vi "Validate Line Configuration Test.vi"() -> (2 "Pass":bool)   [LabVIEW 2015, in "Modbus Tests.lvlib"]
doc: "Test validate line configuration.vi to ensure that it catches all unique cases in which a channel should not be added to an existing configuration."
uses:
  Modbus Tests.lvlib
  editor node/table line.ctl
  module/module channel/Modbus Module Channel.lvclass
  <vilib>/NI/Tag Bus/tag/Data Type.ctl
  module/module channel/data bank type.ctl
  <vilib>/NI/Tag Bus Module Framework/channel/channel classification.ctl
  module/configuration/Modbus Module configuration.lvclass
  <vilib>/NI/Tag Bus/tag/tag descriptor.lvclass/tag descriptor.ctl
  module/module channel/Modbus Module Channel.lvclass/Modbus Module Channel.ctl
  <vilib>/NI/Tag Bus Module Framework/channel/TBM channel.lvclass/TBM channel.ctl
  <vilib>/NI/Tag Bus/tag/write data type.vi
  <vilib>/NI/Tag Bus/tag/write tag name.vi
  module/module channel/Write modbus type.vi
  module/module channel/Write starting address.vi
  module/module channel/Write subindex (bool).vi
  <vilib>/NI/Tag Bus Module Framework/channel/Write channel classification.vi
  editor node/Modbus Module editor node.lvclass
  <vilib>/NI/Tag Bus/tag/tag descriptor.lvclass
  <vilib>/NI/Tag Bus Module Framework/channel/TBM channel.lvclass
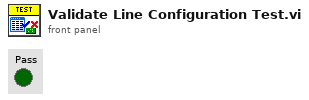
[diagram p1: front panel]
types:
  T1 = typedef "Modbus Module Channel.lvclass/data bank type.ctl" = enum16{"Coils", "Discrete Inputs", "Input Registers", "Holding Registers"}
  T2 = typedef "tag bus.lvlib/tag descriptor.lvclass/Data Type.ctl" = enum16{"Double", "Single", "I64", "I32", "I16", "I8", "U64", "U32", "U16", "U8", "Boolean", "String", "Array of Double", "Array of Single", "Array of I64", "Array of I32", "Array of I16", "Array of I8", "Array of U64", "Array of U32", "Array of U16", "Array of U8", "Array of Boolean", "Array of String"}
  T3 = typedef "TBM channel.lvclass/channel classification.ctl" = enum16{"input data", "output data", "processing parameter", "processing result"}
  T4 = typedef "Modbus Module editor node.lvclass/table line.ctl" = cluster{"mbchan":refnum<class "Modbus Module Channel.lvclass">, "tag name":string}
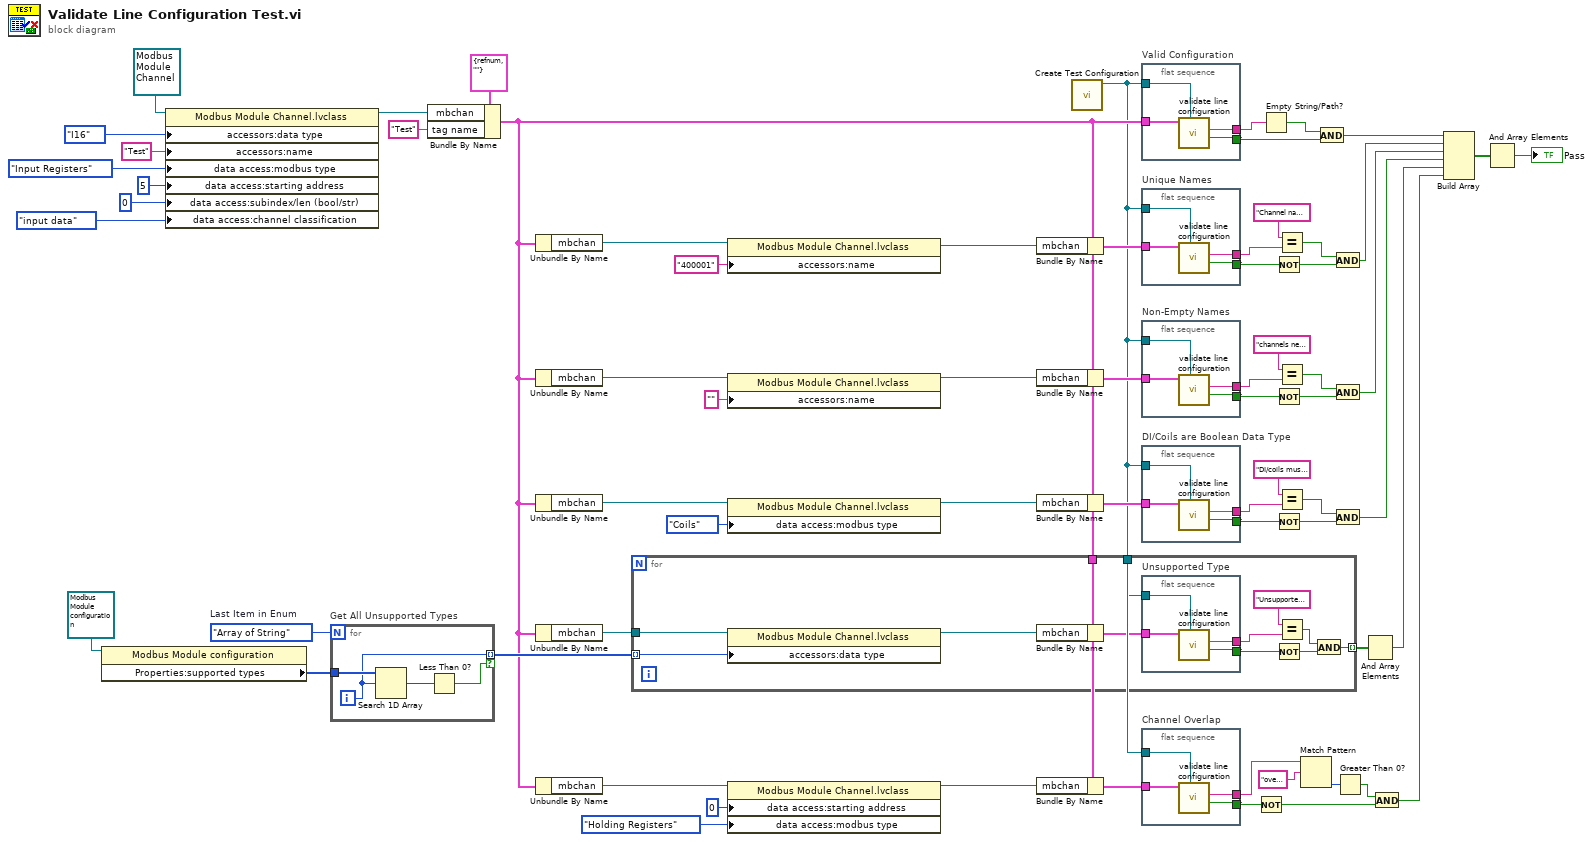
[diagram p0: block diagram]
diagram:
  w17 = Data_Type."Array of String"  # Last Item in Enum
  n1 = property class="Modbus Module configuration"(reference=refnum<class "Modbus Module configuration.lvclass"> refnum ("Modbus Module configuration")) -> ("Properties:supported types"=w18:T2[])  [unwired: 1 in, 2 out]
  n2 = property class="Modbus Module Channel.lvclass"(reference=refnum<class "Modbus Module Channel.lvclass"> refnum ("mbchan"), "accessors:data type"=Data_Type."I16" ("data type"), "accessors:name"="Test" ("name"), "data access:modbus type"=data_bank_type."Input Registers" ("modbus type"), "data access:starting address"=u16 5 ("starting address"), "data access:subindex/len (bool/str)"=0 ("subindex/len (bool/str)"), "data access:channel classification"=channel_classification."input data" ("channel classification")) -> (reference out=w64:refnum<class "Modbus Module Channel.lvclass">)  [unwired: 1 in, 1 out]
  n3 = for "Get All Unsupported Types" {
    N: w17 -> [_]
    tunnel: w18 -> [w71]
    tunnel: [w69] -> w15 mode=indexing if=w68
    i -> [w69]
    n4 = Search 1D Array(1D array=w71, element=w69) -> (index of element=w70:i32)  [unwired: 1 in]
    n5 = Less Than 0?(x=w70) -> (x < 0?=w68:bool)
  }
  n6 = Bundle By Name(cluster=T4 {"mbchan"=refnum, "tag name"=""} ("line in"), "mbchan"=w64, "tag name"="Test") -> (w10:T4)
  n7 = Unbundle By Name(w10) -> ("mbchan"=w51:refnum<class "Modbus Module Channel.lvclass">)
  n8 = Unbundle By Name(w10) -> ("mbchan"=w33:refnum<class "Modbus Module Channel.lvclass">)
  n9 = Unbundle By Name(w10) -> ("mbchan"=w30:refnum<class "Modbus Module Channel.lvclass">)
  n10 = Unbundle By Name(w10) -> ("mbchan"=w21:refnum<class "Modbus Module Channel.lvclass">)
  n11 = Unbundle By Name(w10) -> ("mbchan"=w11:refnum<class "Modbus Module Channel.lvclass">)
  n12 = property class="Modbus Module Channel.lvclass"(reference=w51, "accessors:name"="400001" ("name")) -> (reference out=w49:refnum<class "Modbus Module Channel.lvclass">)  [unwired: 1 in, 1 out]
  n13 = property class="Modbus Module Channel.lvclass"(reference=w33, "accessors:name"="" ("name")) -> (reference out=w32:refnum<class "Modbus Module Channel.lvclass">)  [unwired: 1 in, 1 out]
  n14 = property class="Modbus Module Channel.lvclass"(reference=w30, "data access:modbus type"=data_bank_type."Coils" ("modbus type")) -> (reference out=w31:refnum<class "Modbus Module Channel.lvclass">)  [unwired: 1 in, 1 out]
  n15 = property class="Modbus Module Channel.lvclass"(reference=w11, "data access:starting address"=u16 0 ("starting address"), "data access:modbus type"=data_bank_type."Holding Registers" ("modbus type")) -> (reference out=w12:refnum<class "Modbus Module Channel.lvclass">)  [unwired: 1 in, 1 out]
  n16 = Bundle By Name(cluster=w10, "mbchan"=w49) -> (w50:T4)
  n17 = Bundle By Name(cluster=w10, "mbchan"=w32) -> (w36:T4)
  n18 = Bundle By Name(cluster=w10, "mbchan"=w31) -> (w29:T4)
  n19 = Bundle By Name(cluster=w10, "mbchan"=w12) -> (w13:T4)
  n20 = call "Create Test Configuration.vi"() -> ("Module configuration"=w9:refnum<class "Modbus Module configuration.lvclass">)  [unwired: 8 in, 3 out]
  n21 = for {
    tunnel: w21 -> [w77]
    tunnel: w10 -> [w75]
    tunnel: w9 -> [w74]
    tunnel: [w73] -> w19 mode=indexing
    tunnel: w15 -> [w72] mode=indexing
    n22 = property class="Modbus Module Channel.lvclass"(reference=w77, "accessors:data type"=w72) -> (reference out=w76:refnum<class "Modbus Module Channel.lvclass">)  [unwired: 1 in, 1 out]
    n23 = Bundle By Name(cluster=w75, "mbchan"=w76) -> (w78:T4)
    n24 = flat-sequence "Unsupported Type" {
      tunnel: w78 -> [w87]
      tunnel: [w86] -> w80
      tunnel: [w85] -> w79
      tunnel: w74 -> [w84]
      frame #0 {
        n25 = call "validate line configuration.vi"("modbus"=w84, "line in"=w87) -> ("valid?"=w85:bool, "issues"=w86:string)  [unwired: 7 in, 1 out]
      }
    }
    n26 = Not(x=w79) -> (.not. x?=w83:bool)
    n27 = Equal?(x="Unsupported type", y=w80) -> (x = y?=w81:bool)
    n28 = And(x=w81, y=w83) -> (x .and. y?=w73:bool)
  }
  n29 = flat-sequence "Valid Configuration" {
    tunnel: w10 -> [w91]
    tunnel: [w90] -> w57
    tunnel: [w89] -> w55
    tunnel: w9 -> [w88]
    frame #0 {
      n30 = call "validate line configuration.vi"("modbus"=w88, "line in"=w91) -> ("valid?"=w89:bool, "issues"=w90:string)  [unwired: 7 in, 1 out]
    }
  }
  n31 = flat-sequence "Unique Names" {
    tunnel: w50 -> [w95]
    tunnel: [w94] -> w46
    tunnel: [w93] -> w47
    tunnel: w9 -> [w92]
    frame #0 {
      n32 = call "validate line configuration.vi"("modbus"=w92, "line in"=w95) -> ("valid?"=w93:bool, "issues"=w94:string)  [unwired: 7 in, 1 out]
    }
  }
  n33 = flat-sequence "Non-Empty Names" {
    tunnel: w36 -> [w99]
    tunnel: [w98] -> w38
    tunnel: [w97] -> w37
    tunnel: w9 -> [w96]
    frame #0 {
      n34 = call "validate line configuration.vi"("modbus"=w96, "line in"=w99) -> ("valid?"=w97:bool, "issues"=w98:string)  [unwired: 7 in, 1 out]
    }
  }
  n35 = flat-sequence "DI/Coils are Boolean Data Type" {
    tunnel: w29 -> [w103]
    tunnel: [w102] -> w27
    tunnel: [w101] -> w28
    tunnel: w9 -> [w100]
    frame #0 {
      n36 = call "validate line configuration.vi"("modbus"=w100, "line in"=w103) -> ("valid?"=w101:bool, "issues"=w102:string)  [unwired: 7 in, 1 out]
    }
  }
  n37 = flat-sequence "Channel Overlap" {
    tunnel: w13 -> [w104]
    tunnel: [w107] -> w2
    tunnel: [w106] -> w14
    tunnel: w9 -> [w105]
    frame #0 {
      n38 = call "validate line configuration.vi"("modbus"=w105, "line in"=w104) -> ("valid?"=w106:bool, "issues"=w107:string)  [unwired: 7 in, 1 out]
    }
  }
  n39 = Not(x=w14) -> (.not. x?=w8:bool)
  n40 = Empty String/Path?(string/path=w57) -> (empty?=w56:bool)
  n41 = Not(x=w47) -> (.not. x?=w43:bool)
  n42 = Not(x=w37) -> (.not. x?=w41:bool)
  n43 = Not(x=w28) -> (.not. x?=w24:bool)
  n44 = Equal?(x="Channel name must be unique", y=w46) -> (x = y?=w45:bool)
  n45 = Equal?(x="channels need a name", y=w38) -> (x = y?=w39:bool)
  n46 = Equal?(x="DI/coils must be boolean", y=w27) -> (x = y?=w26:bool)
  n47 = Match Pattern(string=w2, regular expression="overlaps with this channel") -> (offset past match=w4:i32)  [unwired: 1 in, 3 out]
  n48 = And(x=w56, y=w55) -> (x .and. y?=w54:bool)
  n49 = And(x=w45, y=w43) -> (x .and. y?=w42:bool)
  n50 = And(x=w39, y=w41) -> (x .and. y?=w35:bool)
  n51 = And(x=w26, y=w24) -> (x .and. y?=w23:bool)
  n52 = Greater Than 0?(x=w4) -> (x > 0?=w3:bool)
  n53 = And Array Elements(Boolean array=w19) -> (logical AND=w16:bool)
  n54 = And(x=w3, y=w8) -> (x .and. y?=w7:bool)
  n55 = Build Array(w54, w42, w35, w23, w16, w7) -> (w53:bool[])
  n56 = And Array Elements(Boolean array=w53) -> (logical AND=→"Pass":bool)
